vi "Sec Velocities.vi"(0 "NDHX Tube Diameter (m)":dbl, 1 "Sec Cold Density (kg/m^3)":dbl, 2 "Sec Hot Density (kg/m^3) in":dbl, 3 "Sec Ave Density (kg/m^3) 3":dbl, 5 "NDHX Number of Tubes":dbl, 7 "Sec Mass Flow (kg/s)":dbl, 9 "MHX Tube Diameter (m)":dbl, 12 "MHX Tube Pitch (m)":dbl, 13 "Pipe XArea (m^2)":dbl, 14 "Dctl (m)":dbl) -> (4 "Shell Crossflow Area (m^2)":dbl, 6 "Sec Cold Velocity (m/s)":dbl, 8 "Sec Hot Velocity (m/s)":dbl, 10 "Sec MHX Velocity (m/s)":dbl, 15 "Sec NDHX Velocity (m/s)":dbl)   [LabVIEW 2019]
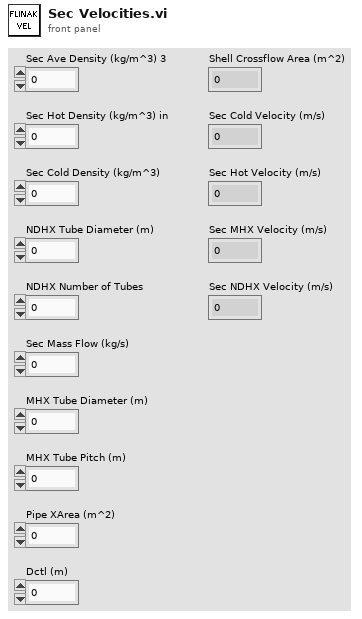
[diagram p1: front panel]
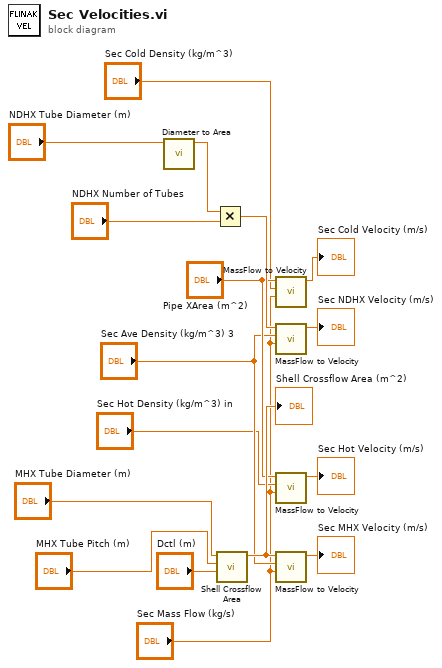
[diagram p0: block diagram]
diagram:
  n1 = call "Diameter to Area.vi"("Diameter (m)"="NDHX Tube Diameter (m)") -> ("Area (m^2)"=w16:dbl)  [unwired: 10 in]
  n2 = Multiply(x=w16, y="NDHX Number of Tubes") -> (x*y=w17:dbl)
  n3 = call "Shell Crossflow Area.vi"("Dctl (m)"="Dctl (m)", "MHX Tube Pitch (m)"="MHX Tube Pitch (m)", "MHX Tube Diameter (m)"="MHX Tube Diameter (m)") -> ("Shell Crossflow Area (m^2)"=w13:dbl)  [unwired: 8 in]
  "Shell Crossflow Area (m^2)" <- w13
  n4 = call "MassFlow to Velocity.vi"("Mass Flow (kg/s)"="Sec Mass Flow (kg/s)", "Density (kg/m^3)"="Sec Cold Density (kg/m^3)", "Area (m^2)"="Pipe XArea (m^2)") -> ("Velocity (m/s)"=→"Sec Cold Velocity (m/s)":dbl)  [unwired: 8 in]
  n5 = call "MassFlow to Velocity.vi"("Mass Flow (kg/s)"="Sec Mass Flow (kg/s)", "Density (kg/m^3)"="Sec Ave Density (kg/m^3) 3", "Area (m^2)"=w17) -> ("Velocity (m/s)"=→"Sec NDHX Velocity (m/s)":dbl)  [unwired: 8 in]
  n6 = call "MassFlow to Velocity.vi"("Mass Flow (kg/s)"="Sec Mass Flow (kg/s)", "Density (kg/m^3)"="Sec Hot Density (kg/m^3) in", "Area (m^2)"="Pipe XArea (m^2)") -> ("Velocity (m/s)"=→"Sec Hot Velocity (m/s)":dbl)  [unwired: 8 in]
  n7 = call "MassFlow to Velocity.vi"("Mass Flow (kg/s)"="Sec Mass Flow (kg/s)", "Density (kg/m^3)"="Sec Ave Density (kg/m^3) 3", "Area (m^2)"=w13) -> ("Velocity (m/s)"=→"Sec MHX Velocity (m/s)":dbl)  [unwired: 8 in]
